vi "Create Combined Graph.vi"(0 "Headers":cluster{string[]}[](array[cluster]), 5 "Data":cluster{dbl[][]}[](array[cluster]), 9 "Axis Select Array":string[](array[string])) -> (6 "Graph":cluster{dbl[], dbl[]}[](array[cluster]))   [LabVIEW 2019]
panel:
  out "XY Graph":cluster{dbl[], dbl[]}[](graph)
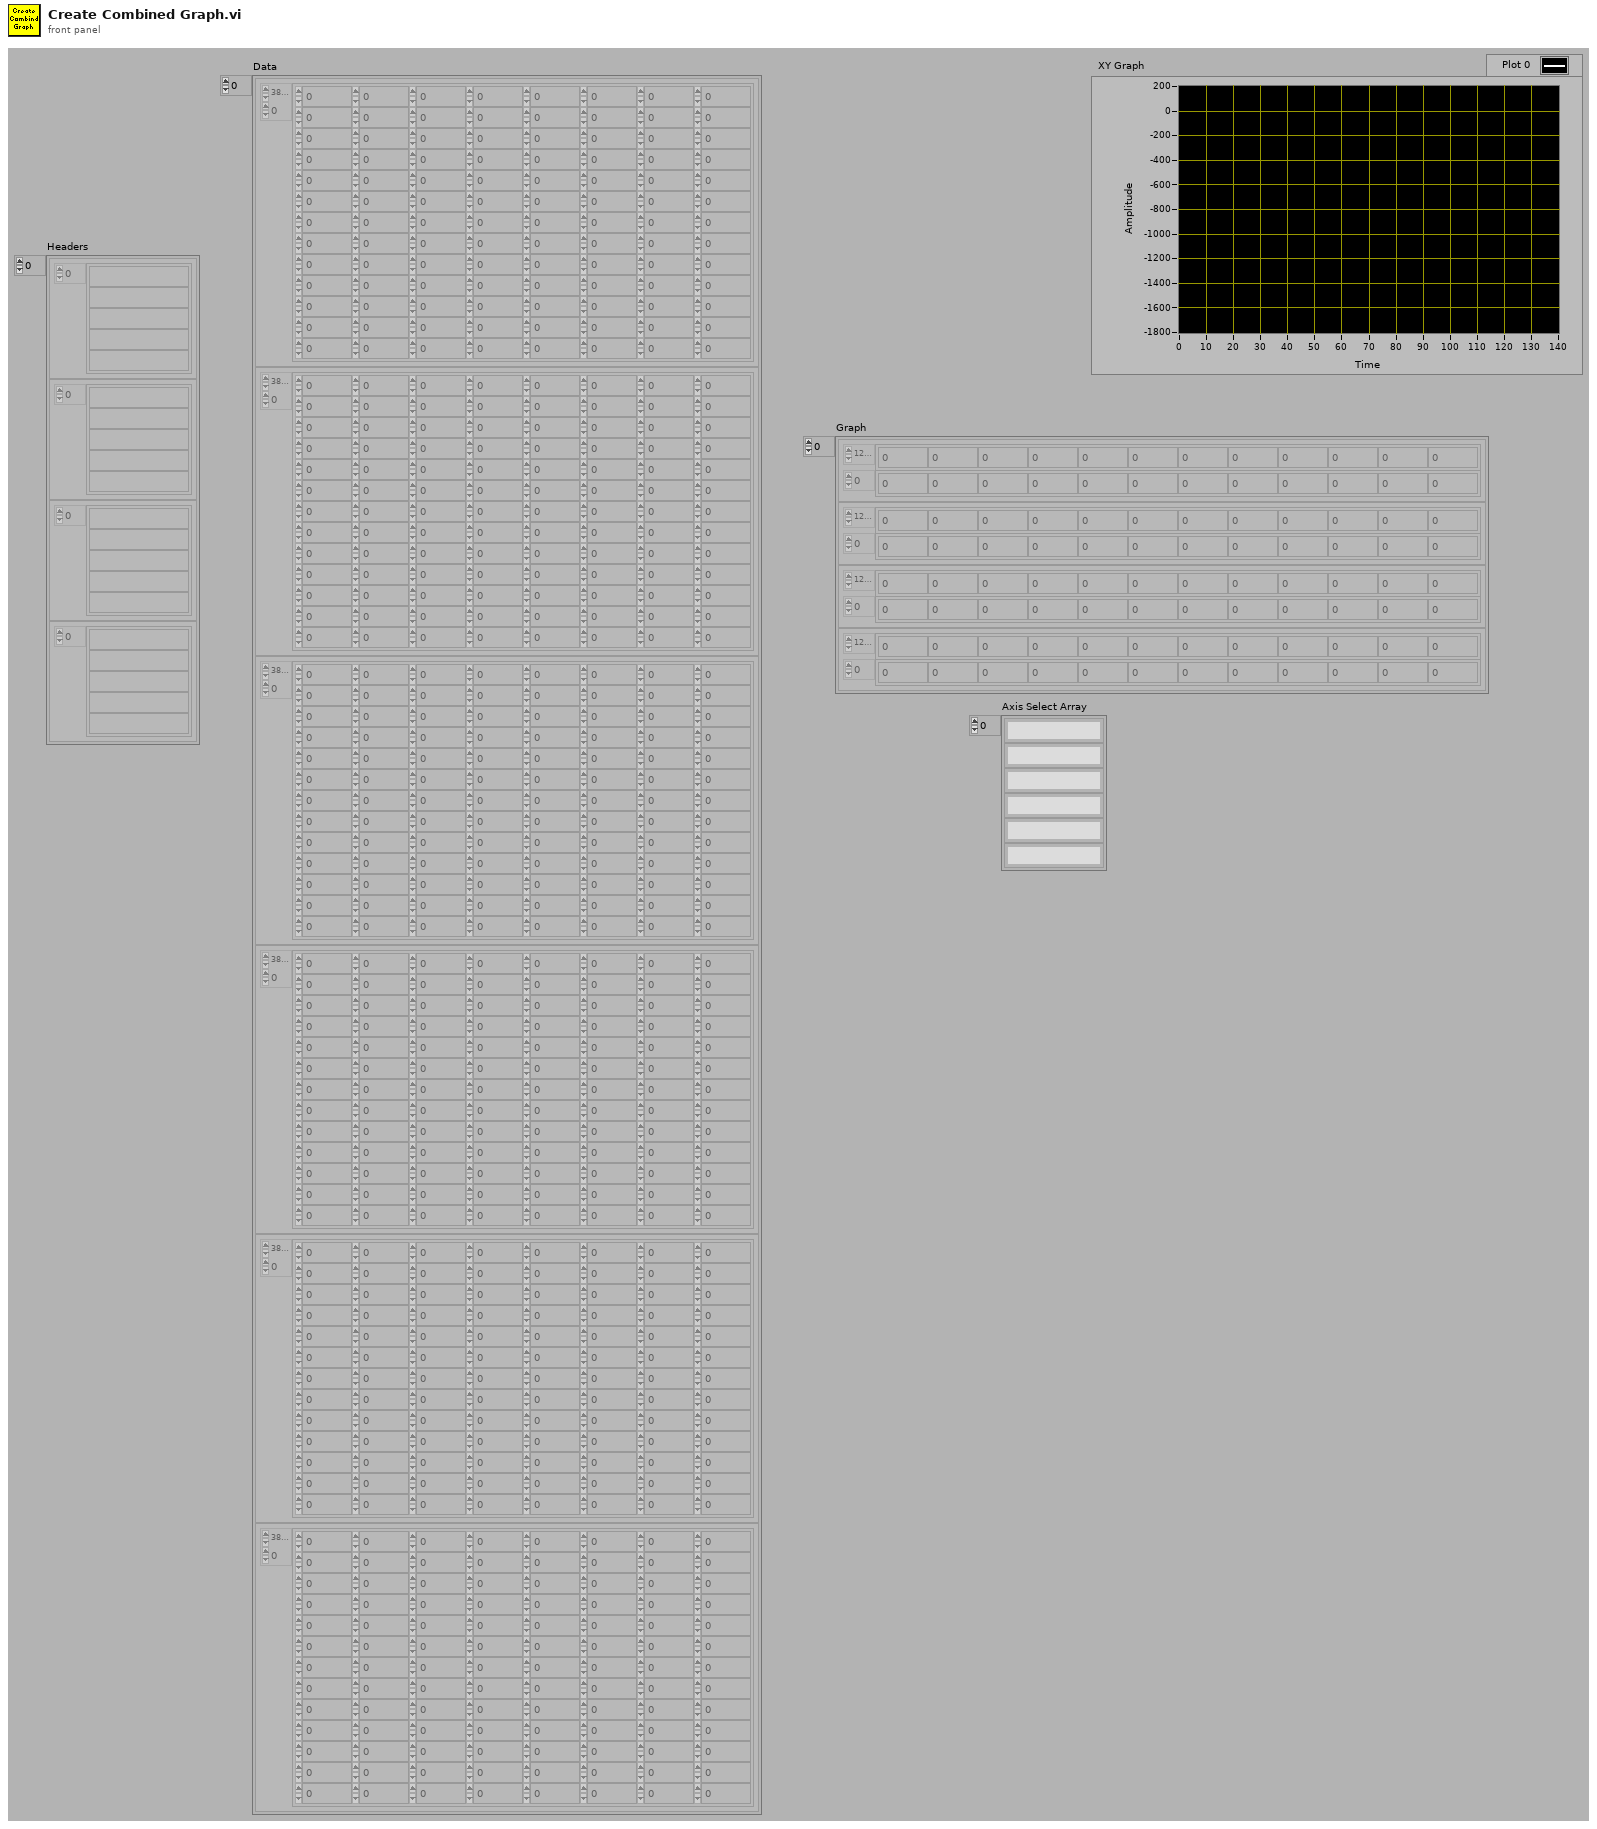
[diagram p1: front panel]
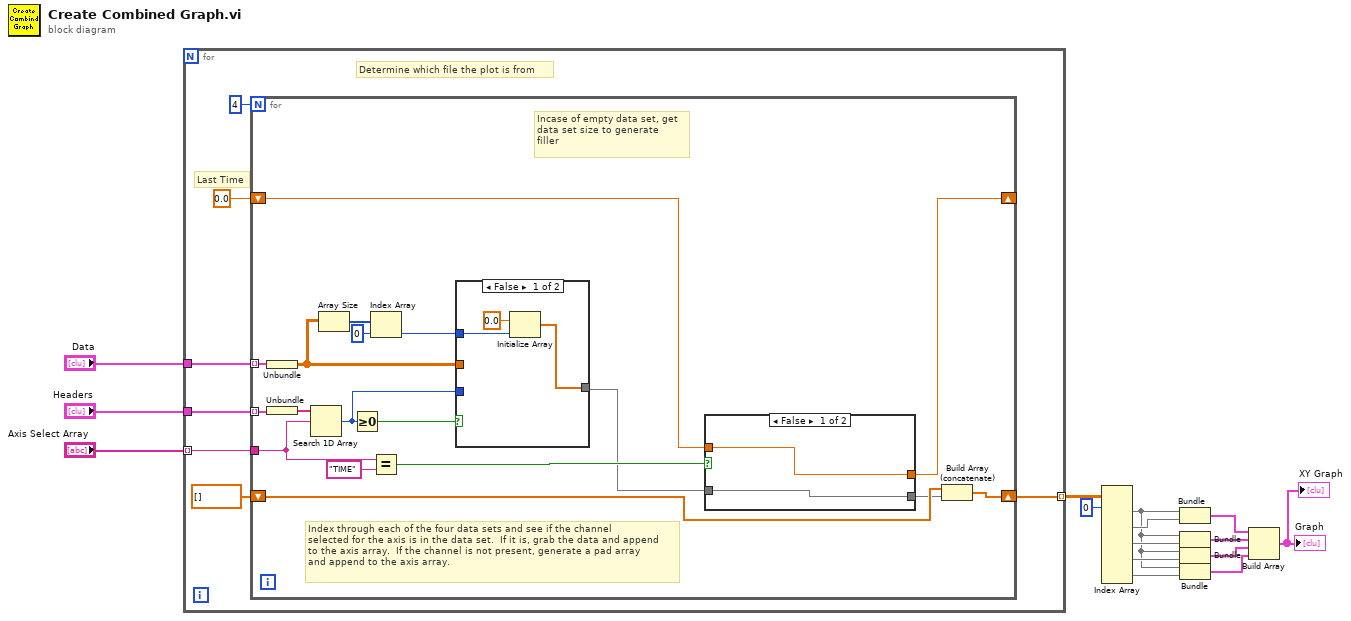
[diagram p0: block diagram]
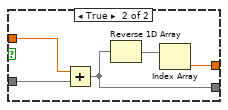
[diagram p2: hidden frame]
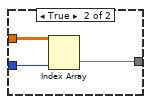
[diagram p3: hidden frame]
diagram:
  n1 = for {
    tunnel: "Data" -> [w20]
    tunnel: "Headers" -> [w21]
    tunnel: "Axis Select Array" -> [w22] mode=indexing
    tunnel: [w18] -> w2 mode=indexing
    # "Last Time"
    # "Determine which file the plot is from"
    n2 = for {
      N: 4 -> [_]
      tunnel: w22 -> [w31]
      tunnel: w21 -> [w40] mode=indexing
      tunnel: w20 -> [w38] mode=indexing
      shift-right: [w25] -> w18
      shift-left: dbl[] [] -> [w24]
      shift-right: [w27] -> _
      shift-left: 0.0 -> [w28]
      # "Index through each of the four data sets and see if the channel\nselected for the axis is in the data set.  If it is, grab the data and append\nto the axis array.  If the channel is not present, generate a pad array\nand append to the axis array."
      # "Incase of empty data set, get\ndata set size to generate\nfiller"
      n3 = Unbundle(w38) -> (w33:dbl[][])
      n4 = Unbundle(w40) -> (w39:string[])
      n5 = Search 1D Array(1D array=w39, element=w31) -> (index of element=w32:i32)  [unwired: 1 in]
      n6 = Array Size(array=w33) -> (size(s)=w37:i32[])
      n7 = Greater Or Equal To 0?(x=w32) -> (x >= 0?=w35:bool)
      n8 = Index Array(array=w37, index=0) -> (element=w34:i32)
      n9 = Equal?(x=w31, y="TIME") -> (x = y?=w29:bool)
      n10 = case shown="False" w35 {
        tunnel: w34 -> [w50 _]
        tunnel: w33 -> [_ w53]
        tunnel: w32 -> [_ w52]
        tunnel: [w48 w51] -> w26
        frame False {
          n11 = Initialize Array(0.0 ("element"), w50) -> (w48:dbl[])
        }
        frame True {
          n12 = Index Array(array=w53, index (col)=w52) -> (element=w51:dbl[])  [unwired: 1 in]
        }
      }
      n13 = case shown="False" w29 {
        tunnel: w26 -> [w41 w47]
        tunnel: [w41 w45] -> w23
        tunnel: w28 -> [w42 w46]
        tunnel: [w42 w43] -> w27
        frame False {
        }
        frame True {
          n14 = Add(x=w46, y=w47) -> (x+y=w45:dbl[])
          n15 = Reverse 1D Array(array=w45) -> (reversed array=w44:dbl[])
          n16 = Index Array(array=w44) -> (element=w43:dbl)  [unwired: 1 in]
        }
      }
      n17 = Build Array (concatenate)(w24, w23) -> (w25:dbl[])
    }
  }
  n18 = Index Array(array=w2, index (row) #1=0 ("index (row)")) -> (element #1=w1:dbl[], element #2=w8:dbl[], element #3=w11:dbl[], element #4=w10:dbl[], element #5=w9:dbl[])  [unwired: 9 in]
  n19 = Bundle(w1, w8) -> (w7:cluster{dbl[], dbl[]})  [unwired: 1 in]
  n20 = Bundle(w1, w11) -> (w6:cluster{dbl[], dbl[]})  [unwired: 1 in]
  n21 = Bundle(w1, w10) -> (w5:cluster{dbl[], dbl[]})  [unwired: 1 in]
  n22 = Bundle(w1, w9) -> (w4:cluster{dbl[], dbl[]})  [unwired: 1 in]
  n23 = Build Array(w7, w6, w5, w4) -> (→"Graph" →"XY Graph":cluster{dbl[], dbl[]}[])
